vi "RoboBees_ArcSin_using_Taylor_Series_Expansion_w_Help.vi"() -> ()   [LabVIEW 2015]
panel:
  out "Time to run":dbl
  out "Angle (Radians)":dbl
  in  "Sin Input\n0 to 1":dbl format="%#_31g"
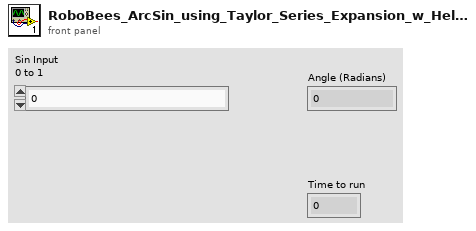
[diagram p1: front panel]
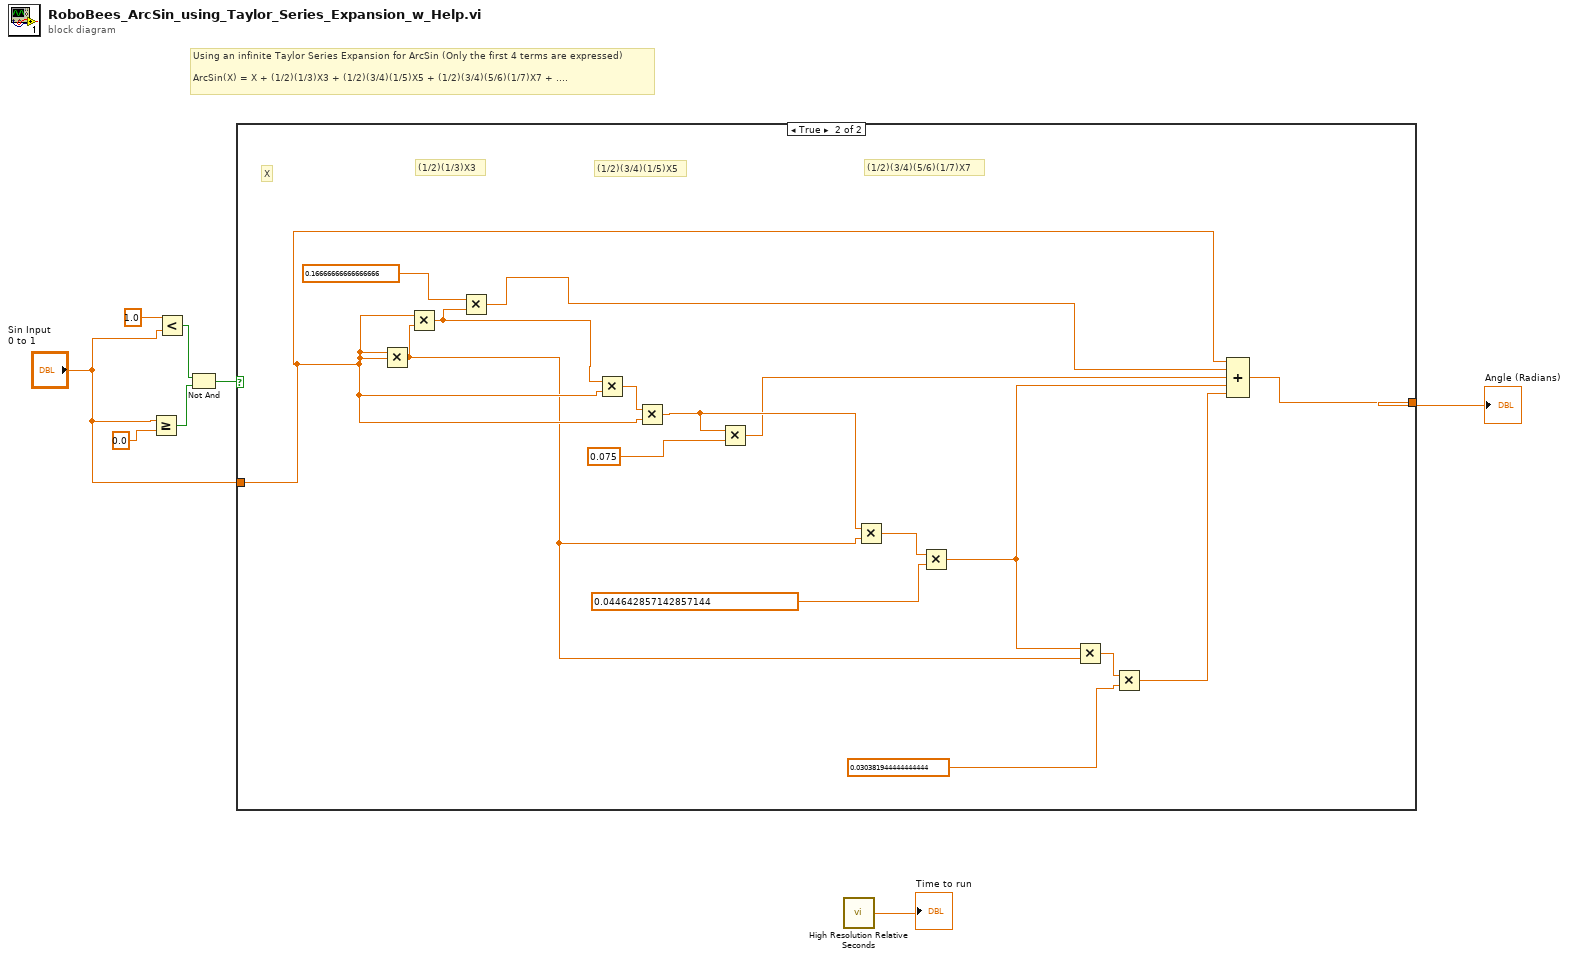
[diagram p0: block diagram]
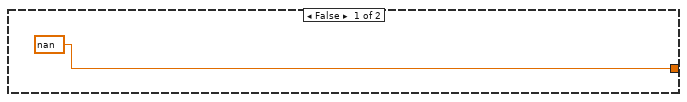
[diagram p2: hidden frame]
diagram:
  # "Using an infinite Taylor Series Expansion for ArcSin (Only the first 4 terms are expressed)\n\nArcSin(X) = X + (1/2)(1/3)X3 + (1/2)(3/4)(1/5)X5 + (1/2)(3/4)(5/6)(1/7)X7 + ...."
  n1 = Greater Or Equal?(x="Sin Input\n0 to 1", y=0.0) -> (x >= y?=w1:bool)
  n2 = Less?(x=1.0, y="Sin Input\n0 to 1") -> (x < y?=w2:bool)
  n3 = Not And(1:w1, 2:w2) -> (0:w3:bool)
  n4 = case shown="True" w3 {
    tunnel: [nan w17] -> w8
    tunnel: "Sin Input\n0 to 1" -> [_ w15]
    frame False {
    }
    frame True {
      # "(1/2)(3/4)(5/6)(1/7)X7"
      # "(1/2)(3/4)(1/5)X5"
      # "(1/2)(1/3)X3"
      # "X"
      n5 = Multiply(x=w15, y=w15) -> (x*y=w13:dbl)
      n6 = Multiply(x=w15, y=w13) -> (x*y=w24:dbl)
      n7 = Multiply(x=0.16666666666666666, y=w24) -> (x*y=w16:dbl)
      n8 = Multiply(x=w24, y=w15) -> (x*y=w23:dbl)
      n9 = Multiply(x=w23, y=w15) -> (x*y=w21:dbl)
      n10 = Multiply(x=w21, y=0.075) -> (x*y=w18:dbl)
      n11 = Multiply(x=w21, y=w13) -> (x*y=w20:dbl)
      n12 = Multiply(x=w20, y=0.044642857142857144) -> (x*y=w14:dbl)
      n13 = Multiply(x=w14, y=w13) -> (x*y=w12:dbl)
      n14 = Multiply(x=w12, y=0.030381944444444444) -> (x*y=w10:dbl)
      n15 = Compound Arithmetic op=ADD(w15, w16, w18, w14, w10) -> (w17:dbl)
    }
  }
  "Angle (Radians)" <- w8
  n16 = call <vilib>:"High Resolution Relative Seconds.vi"() -> ("relative seconds"=→"Time to run":dbl)
